vi "stopEventsSD.vi"(1 "error in (no error)":errorcluster, 2 "control registration ref":refnum<event-registration>, 3 "Stop event":refnum<event-registration>) -> (0 "error out":errorcluster)   [LabVIEW 2015]
uses:
  Classes/Experiment.lvclass
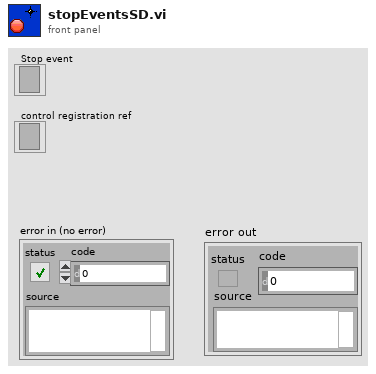
[diagram p1: front panel]
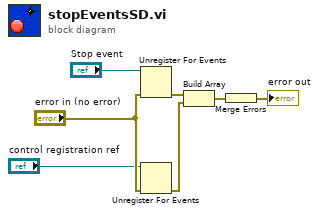
[diagram p0: block diagram]
diagram:
  n1 = Unregister For Events(event registration refnum="Stop event", error in="error in (no error)") -> (error out=w4:errorcluster)
  n2 = Unregister For Events(event registration refnum="control registration ref", error in="error in (no error)") -> (error out=w5:errorcluster)
  n3 = Build Array(w4, w5) -> (w6:errorcluster[])
  n4 = Merge Errors(w6) -> (→"error out":errorcluster)
